vi "GlobalSTATE.vi"() -> ()   [LabVIEW 2021]
panel:
  out "Current State":string="CHOICE"
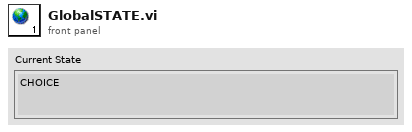
[diagram p1: front panel]
diagram:
